vi "trivial.vi"(0 "Client time":dbl format="%.2f") -> (1 "Server time":dbl format="%.2f", 2 "Difference":dbl format="%.2f")   [LabVIEW 2010]
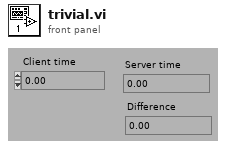
[diagram p1: front panel]
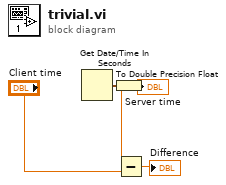
[diagram p0: block diagram]
diagram:
  n1 = Get Date/Time In Seconds() -> (seconds since 1Jan1904=w1:timestamp)
  n2 = To Double Precision Float(number=w1) -> (double precision float=w4:dbl)
  "Server time" <- w4
  n3 = Subtract(x=w4, y="Client time") -> (x-y=→"Difference":dbl)
